vi "Forward For Time.vi"(7 "drive.lvclass":refnum<class "drive.lvclass">, 8 "error in (no error)":errorcluster, 9 "Angle":dbl, 10 "Time (ms)":u32, 11 "Speed":dbl) -> (0 "error out":errorcluster, 3 "drive.lvclass":refnum<class "drive.lvclass">)   [LabVIEW 2015, in "drive.lvclass"]
uses:
  drive.lvclass
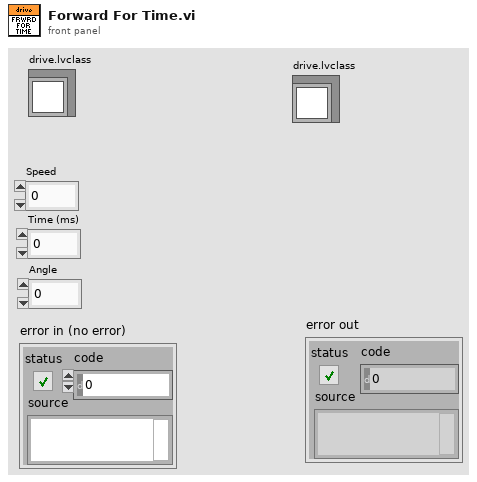
[diagram p1: front panel]
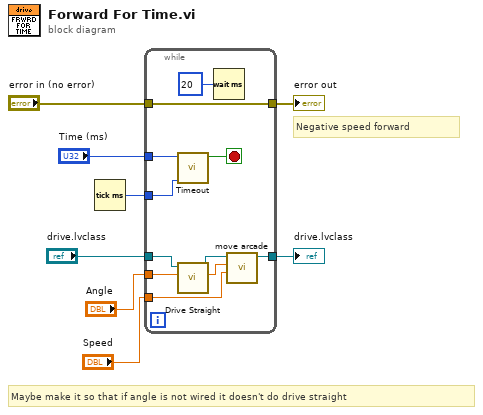
[diagram p0: block diagram]
diagram:
  # "Maybe make it so that if angle is not wired it doesn't do drive straight"
  # "Negative speed forward"
  n1 = Tick Count (ms)() -> (millisecond timer value=w4:u32)
  n2 = while {
    tunnel: "drive.lvclass" -> [w10]
    tunnel: [w16] -> w3
    tunnel: w4 -> [w18]
    tunnel: "Angle" -> [w15]
    tunnel: "Speed" -> [w14]
    tunnel: "Time (ms)" -> [w12]
    tunnel: "error in (no error)" -> [w11]
    tunnel: [w11] -> w1
    stop <- w17 stop-if-true
    n3 = call "Timeout.vi"("Start Time In"=w18, "Time Limit"=w12) -> ("Timeout"=w17:bool)  [unwired: 8 in, 1 out]
    n4 = call "Drive Straight.vi"("Angle robot facing"=w15, "drive.lvclass"=w10) -> ("Arcade drive x"=w13:dbl, "drive.lvclass"=w9:refnum<class "drive.lvclass">)  [unwired: 8 in]
    n5 = Wait (ms)(milliseconds to wait=u32 20) -> ()  [unwired: 1 out]
    n6 = call "move arcade.vi"("Forward Value"=w14, "Turn Value"=w13, "drive.lvclass"=w9) -> ("drive.lvclass"=w16:refnum<class "drive.lvclass">)  [unwired: 8 in]
  }
  "drive.lvclass" <- w3
  "error out" <- w1
